vi "Set High Voltage Return and Ground Bond Channel.vi"(6 "Ground Bond Channel (1)":i32=1, 8 "error in (no error)":errorcluster, 9 "Return Channels":i32[](array[numeric]), 10 "High Voltage Channels":i32[](array[numeric]), 11 "VISA resource name":refnum<visa-resource-name>) -> (0 "error out":errorcluster, 3 "VISA resource name out":refnum<visa-resource-name>)   [LabVIEW 2014, in "Associated Research SC6540.lvlib"]
doc: "Switch the ground bond channel and connect the specified channels to high voltage port and return port at the same time."
uses:
  <instrlib>/Associated Research SC6540/Associated Research SC6540.lvlib
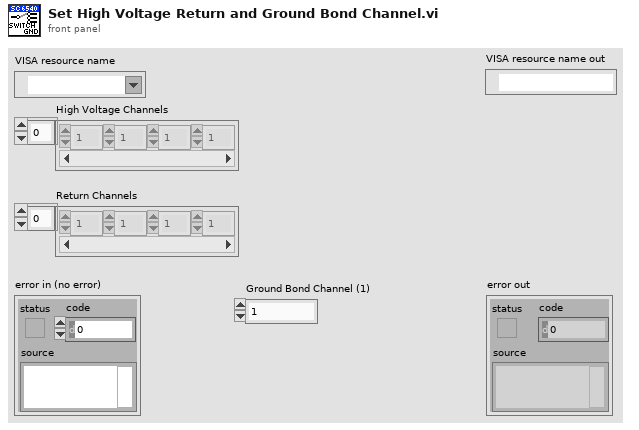
[diagram p1: front panel]
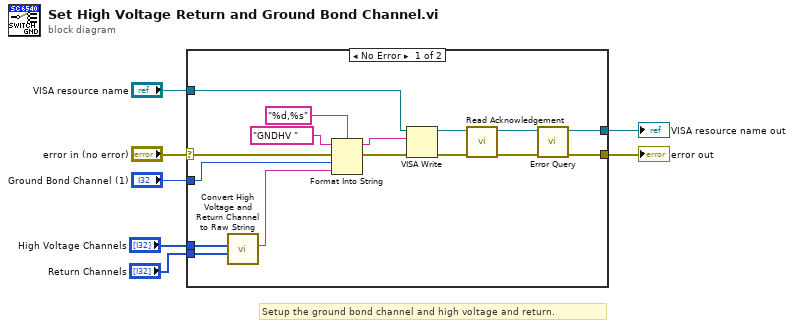
[diagram p0: block diagram]
diagram:
  # "Setup the ground bond channel and high voltage and return."
  n1 = case shown="No Error" "error in (no error)" {
    selector: "error in (no error)" -> [w22 w24]
    tunnel: "Ground Bond Channel (1)" -> [w23 _]
    tunnel: "VISA resource name" -> [w18 w25]
    tunnel: [w12 w25] -> w4
    tunnel: [w11 w24] -> w3
    tunnel: "High Voltage Channels" -> [w10 _]
    tunnel: "Return Channels" -> [w9 _]
    frame No Error {
      n2 = call <instrlib>:"Convert High Voltage and Return Channel to Raw String.vi"("Return Channels"=w9, "High Voltage Channels"=w10) -> ("Command Raw String"=w8:string)  [unwired: 9 in]
      n3 = Format Into String(format string="%d,%s", initial string="GNDHV " ("command"), error in=w22, w23, w8) -> (resulting string=w17:string, error out=w21:errorcluster)
      n4 = VISA Write(VISA resource name=w18, write buffer=w17, error in (no error)=w21) -> (VISA resource name out=w16:refnum<visa-resource-name>, error out=w15:errorcluster)  [unwired: 1 out]
      n5 = call <instrlib>:"Read Acknowledgement.vi"("error in (no error)"=w15, "VISA resource name"=w16) -> ("error out"=w13:errorcluster, "VISA resource name out"=w14:refnum<visa-resource-name>)  [unwired: 8 in]
      n6 = call <instrlib>:"Error Query.vi"("error in (no error)"=w13, "VISA resource name"=w14) -> ("error out"=w11:errorcluster, "VISA resource name out"=w12:refnum<visa-resource-name>)  [unwired: 6 in, 2 out]
    }
    frame Error {
    }
  }
  "VISA resource name out" <- w4
  "error out" <- w3
